vi "SetControlValue.vi"(6 "SIGNAL?":bool, 8 "error in (no error)":errorcluster, 9 "Value":variant, 10 "Control Label":string, 11 "RefCluster In":T1) -> (0 "error out":errorcluster, 3 "RefCluster Out":T1)   [LabVIEW 2020, in "CtlReferences_API.lvlib"]
doc: "Sets the value of the control specified"
uses:
  CtlReferences_API.lvlib
  CtlReferences/CtlReferences.lvclass
  CtlReferences/TypeDefs/CtlLookup.ctl
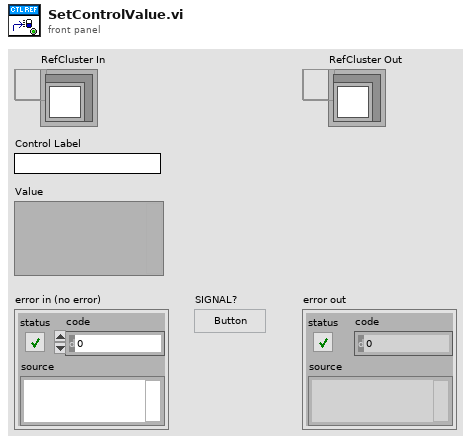
[diagram p1: front panel]
types:
  T1 = typedef "CtlReferences.lvlib/CtlReferences.lvclass/CtlLookup.ctl" = refnum<data-value>
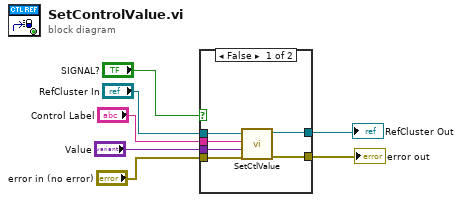
[diagram p0: block diagram]
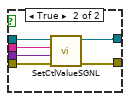
[diagram p2: hidden frame]
diagram:
  n1 = case shown="False" "SIGNAL?" {
    tunnel: [w13 w18] -> w7
    tunnel: [w12 w17] -> w6
    tunnel: "RefCluster In" -> [w11 w19]
    tunnel: "Control Label" -> [w10 w14]
    tunnel: "Value" -> [w9 w15]
    tunnel: "error in (no error)" -> [w8 w16]
    frame False {
      n2 = call "SetCtlValue.vi"("Error in"=w8, "Value"=w9, "CtlName In"=w10, "CtlLookup In"=w11) -> ("error out"=w12:errorcluster, "CtlLookup Out"=w13:T1)  [unwired: 6 in]
    }
    frame True {
      n3 = call "SetCtlValueSGNL.vi"("Error in"=w16, "Value"=w15, "CtlName In"=w14, "CtlLookup In"=w19) -> ("error out"=w17:errorcluster, "CtlLookup Out"=w18:T1)  [unwired: 6 in]
    }
  }
  "RefCluster Out" <- w7
  "error out" <- w6
